vi "_DataType Cacher Core.vi"(0 "key":string, 2 "Type":T1) -> (4 "cacher":variant, 5 "match?":bool, 6 "stored type":T1, 7 "error out":errorcluster)   [LabVIEW 2017]
uses:
  <vilib>/Utility/Data Type/Type Definitions/Data Type.ctl
  431ed5a2-bdaf-49c6-86f1-da6f8952148f.vi
  9126b41d-220b-4c2d-9ba0-52a43fc072d2.vi
  <vilib>/Utility/Data Type/NI_Data Type.lvlib
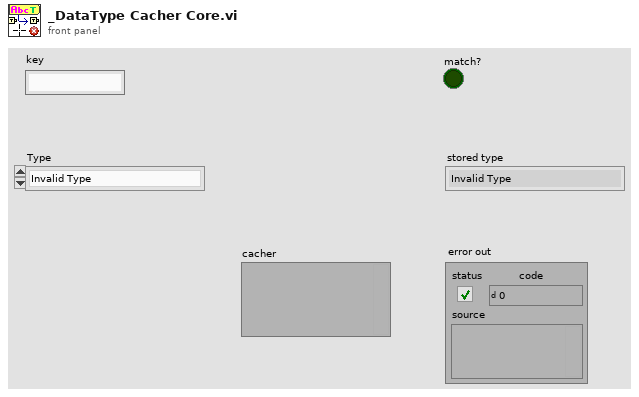
[diagram p1: front panel]
types:
  T1 = typedef "NI_Data Type.lvlib/Data Type.ctl" = enum8{"Invalid Type", "Void", "I8", "I16", "I32", "I64", "U8", "U16", "U32", "U64", "Single Float", "Double Float", "Extended Float", "Single Complex", "Double Complex", "Extended Complex", "Enum U8", "Enum U16", "Enum U32", "Enum U64", "Single Float With Unit", "Double Float With Unit", "Extended Float With Unit", "Single Complex with Unit", "Double Complex with Unit", "Extended Complex with Unit", "Boolean", "String", "Path", "Picture", "Tag", "Array", "Cluster", "Variant", "LV Variant", "Waveform", "Timestamp", "Digital Waveform", "Digital Data", "ExpressData", "Refnum", "External Data", "VI", "Poly VI", "LabVIEW Class Instance", "Fixed Point"}
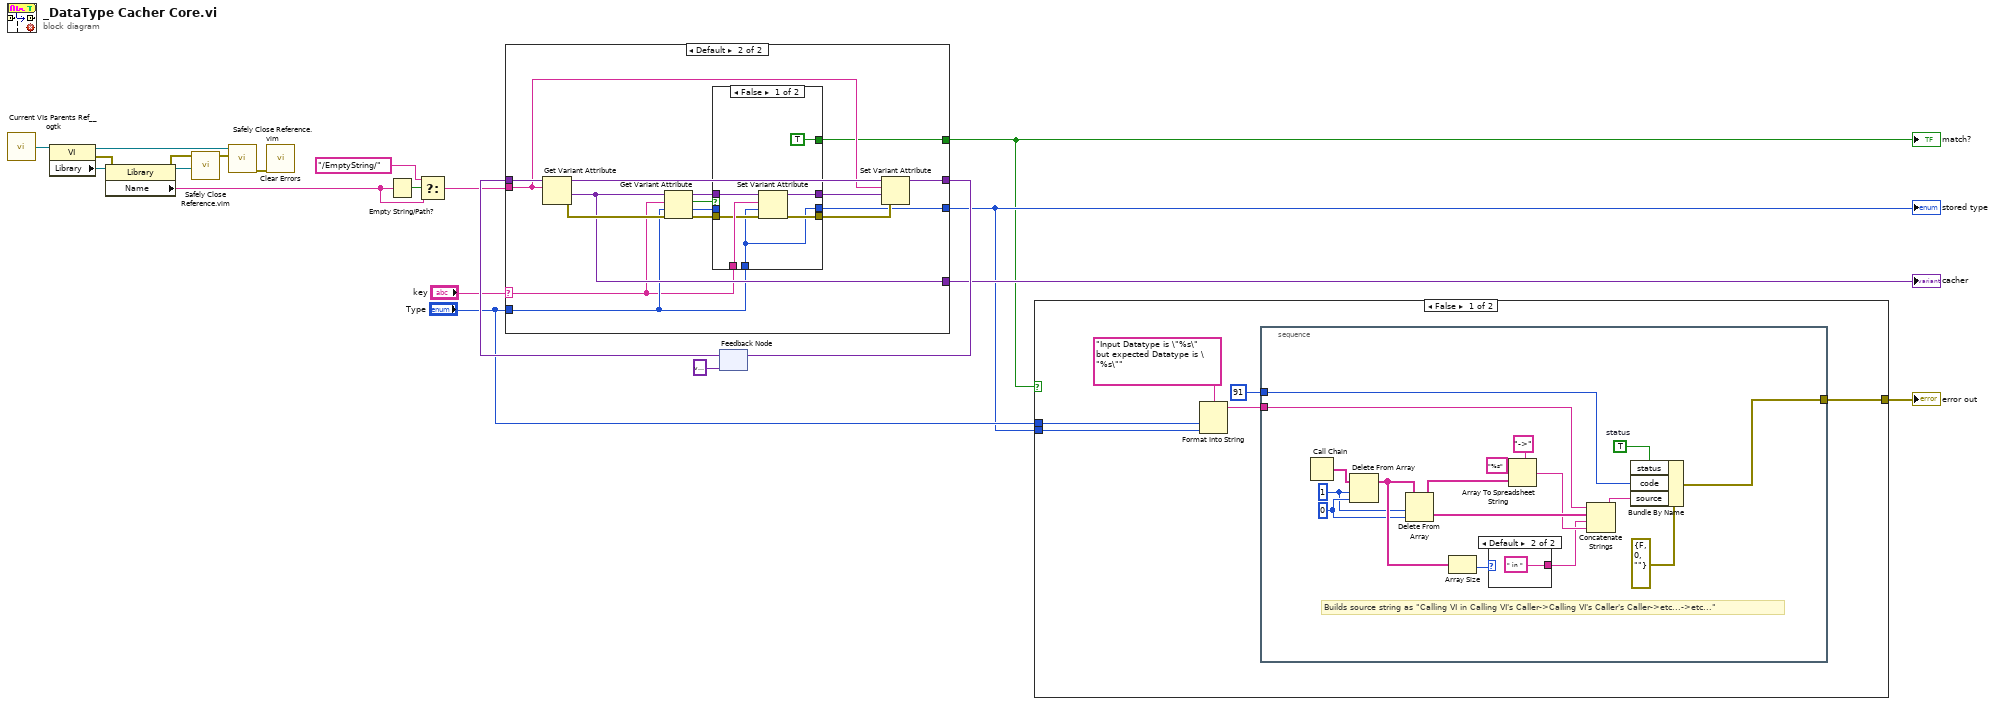
[diagram p0: block diagram]
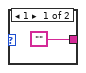
[diagram p2: hidden frame]
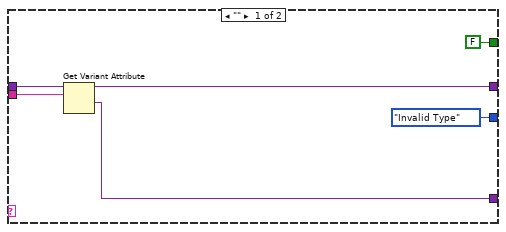
[diagram p4: hidden frame]
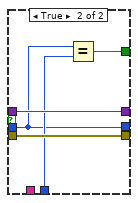
[diagram p5: hidden frame]
diagram:
  n1 = call <userlib>:"Current VIs Parents Ref__ogtk.vi"() -> ("Calling VI's Reference"=w11:refnum<vi>)  [unwired: 2 in]
  n2 = property class="VI"(reference=w11) -> (reference out=w14:refnum<vi>, error out=w13:errorcluster, "Library"=w12:refnum<vi>)  [unwired: 1 in]
  n3 = property class="Library"(reference=w12, error in=w13) -> (reference out=w18:refnum<vi>, error out=w15:errorcluster, "Name"=w20:string)
  n4 = call "Safely Close Reference.vim"("error in (no error)"=w15, "Reference"=w18) -> ("error out"=w17:errorcluster)  [unwired: 9 in]
  n5 = call "Safely Close Reference.vim"("error in (no error)"=w17, "Reference"=w14) -> ("error out"=w16:errorcluster)  [unwired: 9 in]
  n6 = call <vilib>:"Clear Errors.vi"("error in (no error)"=w16) -> ()  [unwired: 5 in, 2 out]
  n7 = Empty String/Path?(string/path=w20) -> (empty?=w19:bool)
  n8 = Select(t="/EmptyString/", s=w19, f=w20) -> (s? t:f=w8:string)
  n9 = feedback #1(variant) -> (w9:variant)
  n10 = case shown="Default" "key" {
    selector: "key" -> [_ w30]
    tunnel: w9 -> [w26 w39]
    tunnel: w8 -> [w27 w36]
    tunnel: [w25 w33] -> w7
    tunnel: [w24 w32] -> w6
    tunnel: "Type" -> [_ w31]
    tunnel: [FALSE w29] -> w1
    tunnel: [Data_Type."Invalid Type" ("Type") w28] -> w2
    frame "" {
      n11 = Get Variant Attribute(Variant=w26, name=w27) -> (duplicate Variant=w25:variant, value=w24:variant)  [unwired: 2 in, 2 out]
    }
    frame Default {
      n12 = Get Variant Attribute(Variant=w39, name=w36) -> (duplicate Variant=w38:variant, value=w32:variant, error out=w35:errorcluster)  [unwired: 2 in, 1 out]
      n13 = Get Variant Attribute(Variant=w32, name=w30, default value (empty Variant)=w31, error in=w35) -> (duplicate Variant=w43:variant, found=w42:bool, value=w41:T1, error out=w40:errorcluster)
      n14 = case shown="False" w42 {
        tunnel: w43 -> [w50 w55]
        tunnel: w30 -> [w49 _]
        tunnel: w41 -> [_ w51]
        tunnel: w40 -> [w48 w54]
        tunnel: [w47 w55] -> w37
        tunnel: [w46 w54] -> w34
        tunnel: w31 -> [w44 w53]
        tunnel: [TRUE w52] -> w29
        tunnel: [w44 w51] -> w28
        frame False {
          n15 = Set Variant Attribute(Variant=w50, name=w49, value=w44, error in=w48) -> (Variant out=w47:variant, error out=w46:errorcluster)  [unwired: 1 out]
        }
        frame True {
          n16 = Equal?(x=w51, y=w53) -> (x = y?=w52:bool)
        }
      }
      n17 = Set Variant Attribute(Variant=w38, name=w36, value=w37, error in=w34) -> (Variant out=w33:variant)  [unwired: 2 out]
    }
  }
  "cacher" <- w6
  "match?" <- w1
  "stored type" <- w2
  n18 = feedback-in #1(w7) -> ()
  n19 = case shown="False" w1 {
    tunnel: [w61 _] -> w4
    tunnel: "Type" -> [w57 _]
    tunnel: w2 -> [w56 _]
    frame False {
      n20 = Format Into String(format string="Input Datatype is \"%s\" but expected Datatype is \"%s\"", w57, w56) -> (resulting string=w58:string)  [unwired: 2 in, 1 out]
      n21 = stacked-sequence {
        tunnel: [w74] -> w61
        tunnel: w58 -> [w75]
        tunnel: 91 ("code") -> [w71]
        frame #0 {
          w68 = 0 ("Index")
          w67 = 1 ("Length")
          w72 = TRUE  # status
          # "Builds source string as \"Calling VI in Calling VI's Caller->Calling VI's Caller's Caller->etc...->etc...\""
          n22 = Call Chain() -> (call chain=w62:string[])
          n23 = Delete From Array(array=w62, length=w67, index=w68) -> (array with subset deleted=w78:string[])  [unwired: 1 out]
          n24 = Delete From Array(array=w78, length=w67, index=w68) -> (deleted portion=w77:string[], array with subset deleted=w69:string[])
          n25 = Array Size(array=w78) -> (size(s)=w76:i32)
          n26 = case shown="Default" w76 {
            tunnel: ["" " in " ("Format String")] -> w64
            frame 1 {
            }
            frame Default {
            }
          }
          n27 = Array To Spreadsheet String(delimiter (Tab)="->", array=w69, 3:"%s" ("format string")) -> (spreadsheet string=w65:string)
          n28 = Concatenate Strings(w75, w77, w64, w65) -> (w73:string)
          n29 = Bundle By Name(cluster=errorcluster {"status"=FALSE, "code"=0, "source"=""} ("error out"), "status"=w72, "code"=w71, "source"=w73) -> (w74:errorcluster)
        }
      }
    }
    frame True {
    }
  }
  "error out" <- w4
